vi "BIO_read_low_level.vi"(8 "error in (no error)":errorcluster, 10 "bytes to read":i32=1024, 11 "BIO in":refnum<class "BIO.lvclass">) -> (0 "error out":errorcluster, 1 "buf":u8[](array[numeric]), 2 "return type":i32, 3 "BIO out":refnum<class "BIO.lvclass">)   [LabVIEW 2013, in "OpenSSL Socket.lvlib" / "BIO.lvclass"]
uses:
  BIO.lvclass
  SSL-Lib/SSL-Lib.lvclass/SSL-Lib.ctl
  BIO.lvclass/BIO.ctl
  SSL-Lib/Read Crypto Library Path.vi
  Read Handle.vi
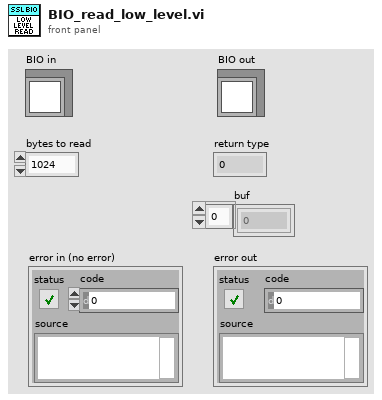
[diagram p1: front panel]
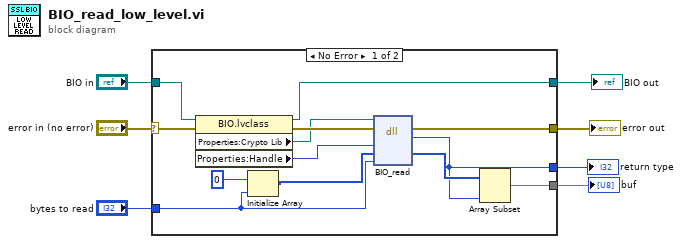
[diagram p0: block diagram]
diagram:
  n1 = case shown="No Error" "error in (no error)" {
    selector: "error in (no error)" -> [w19 w21]
    tunnel: [w20 w21] -> w7
    tunnel: [w9 _] -> w6
    tunnel: "bytes to read" -> [w13 _]
    tunnel: [w8 _] -> w4
    tunnel: "BIO in" -> [w17 w22]
    tunnel: [w15 w22] -> w1
    frame No Error {
      n2 = property class="BIO.lvclass"(reference=w17, error in=w19) -> (reference out=w15:refnum<class "BIO.lvclass">, error out=w18:errorcluster, "Properties:Crypto Lib"=w14:path, "Properties:Handle"=w16:u64)
      n3 = Initialize Array(u8 0, w13) -> (w11:u8[])
      n4 = dll-call lib="C:/Program Files (x86)/National Instruments/Shared/nissl/NIlibeay32.dll" fn="BIO_read"(path in=w14, error in=w18, "BIO"=w16, "buf"=w11, "len"=w13) -> (error out=w20:errorcluster, "return type"=w9:i32, "buf"=w10:u8[])  [unwired: 3 in, 1 out]
      n5 = Array Subset(array=w10, length=w9) -> (w8:u8[])  [unwired: 1 in]
    }
    frame Error {
    }
  }
  "error out" <- w7
  "return type" <- w6
  "buf" <- w4
  "BIO out" <- w1
